vi "Mode.vi"(8 "Error In":errorcluster) -> (0 "Error Out":errorcluster)   [LabVIEW 2017, in "Tests.lvlib" / "Session.lvlib"]
uses:
  Session.lvlib
  src/LabSSH2/Public/Session/Public/Typedefs/Modes.ctl
  src/LabSSH2/Toolkit.lvlib
  src/LabSSH2/Public/Session/Session.lvclass
  <vilib>/addons/_JKI Toolkits/Caraya/classes/Test/Test.lvclass
  <vilib>/addons/_JKI Toolkits/Caraya/classes/Assert/Assert.lvclass
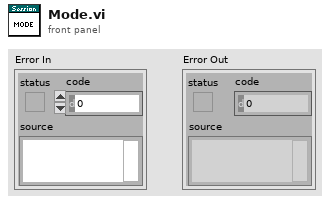
[diagram p1: front panel]
types:
  T1 = typedef "Toolkit.lvlib/Session.lvclass/Modes.ctl" = enum32{"Non-Blocking", "Blocking"}
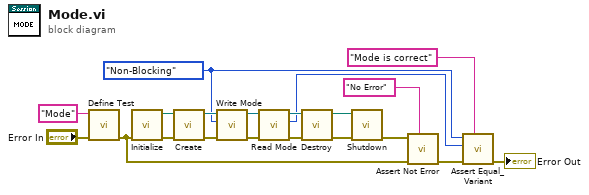
[diagram p0: block diagram]
diagram:
  w2 = Modes."Non-Blocking" ("Mode")
  n1 = call <vilib>:"Define Test.vi"("error in (no error)"="Error In", "Label (VI Title)"="Mode") -> ("error out"=w15:errorcluster)  [unwired: 9 in]
  n2 = call "Initialize.vi"("Error In"=w15) -> ("Error Out"=w19:errorcluster, "labssh2 Shared Library Out"=w12:path)  [unwired: 9 in]
  n3 = call "Create.vi"("Error In"=w19, "labssh2 Shared Library"=w12) -> ("Error Out"=w10:errorcluster, "Sesssion"=w11:refnum<class "Session.lvclass">)  [unwired: 8 in]
  n4 = call "Write Mode.vi"("Error In"=w10, "Mode"=w2, "Session In"=w11) -> ("Error Out"=w9:errorcluster, "Sesssion Out"=w8:refnum<class "Session.lvclass">)  [unwired: 7 in]
  n5 = call "Read Mode.vi"("Error In"=w9, "Session In"=w8) -> ("Error Out"=w6:errorcluster, "Mode"=w1:T1, "Sesssion Out"=w7:refnum<class "Session.lvclass">)  [unwired: 7 in]
  n6 = call "Destroy.vi"("Error In"=w6, "Session"=w7) -> ("Error Out"=w17:errorcluster, "labssh2 Shared Library"=w18:path)  [unwired: 8 in]
  n7 = call "Shutdown.vi"("Error In"=w17, "labssh2 Shared Library"=w18) -> ("Error Out"=w16:errorcluster)  [unwired: 9 in]
  n8 = call <vilib>:"Assert Not Error.vi"("Label"="No Error", "error in (no error)"=w15, "Not Error?"=w16) -> ("error out"=w5:errorcluster)  [unwired: 8 in]
  n9 = call <vilib>:"Assert Equal_Variant.vi"("Label"="Mode is correct", "error in (no error)"=w5, "Y"=w1, "X"=w2) -> ("error out"=→"Error Out":errorcluster)  [unwired: 7 in]
